vi "HV Enclosure test.vi"() -> (0 "HV Enclosure OK":bool)   [LabVIEW 2015]
uses:
  <vilib>/DAQmx/write.llb/DAQmx Write (Digital Bool 1Line 1Point).vi
  <vilib>/DAQmx/read.llb/DAQmx Read (Digital Bool 1Line 1Point).vi
  <vilib>/DAQmx/miscellaneous.llb/DAQmx Fill In Error Info.vi
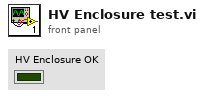
[diagram p1: front panel]
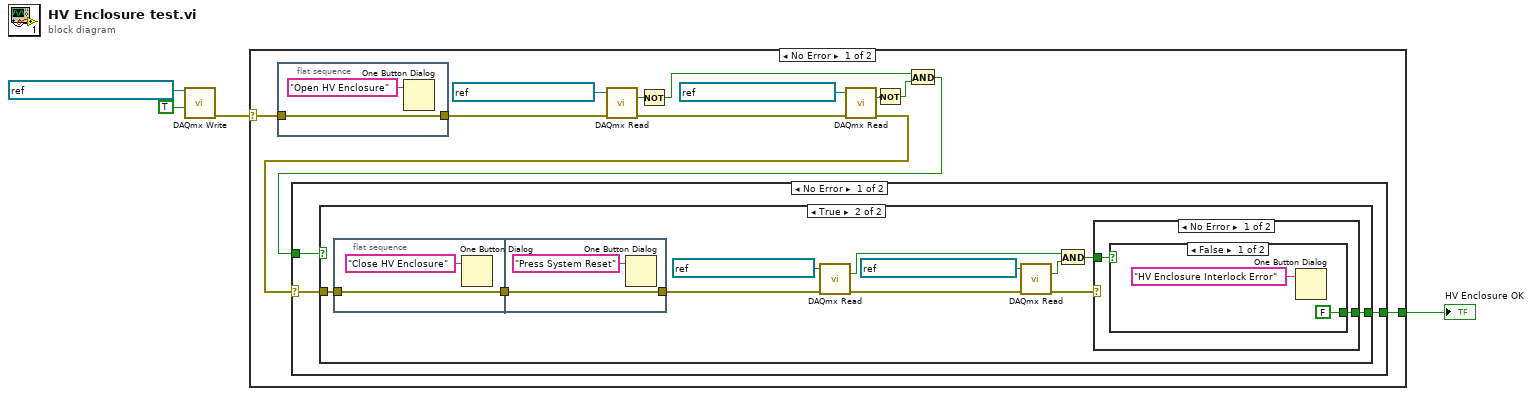
[diagram p0: block diagram]
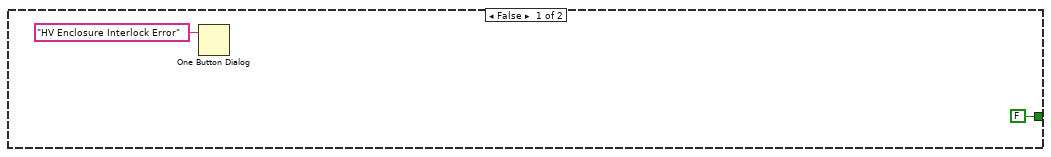
[diagram p2: hidden frame]
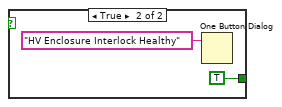
[diagram p3: hidden frame]
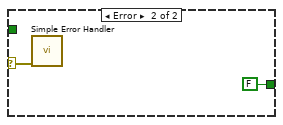
[diagram p4: hidden frame]
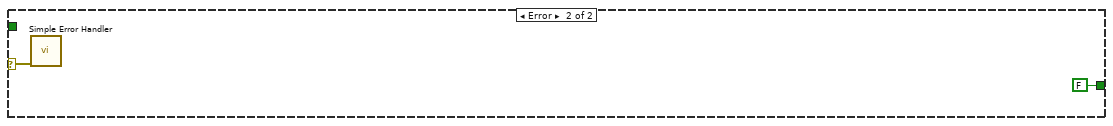
[diagram p5: hidden frame]
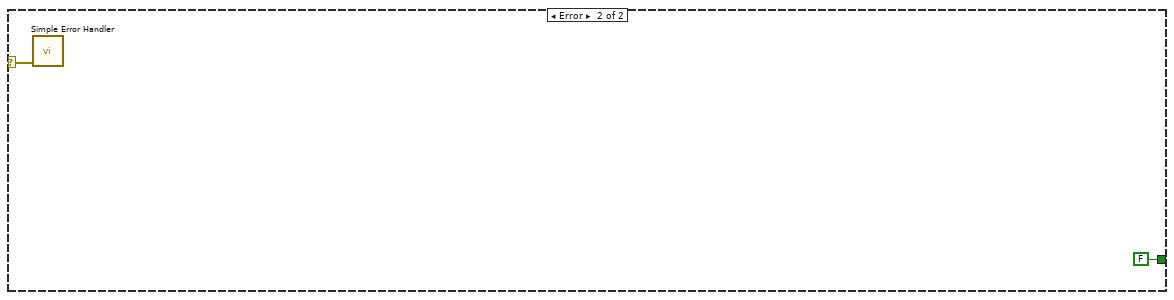
[diagram p6: hidden frame]
diagram:
  n1 = call-poly <vilib>:"DAQmx Write.vi"("task/channels in"=refnum<k21> "DO7 Unlock Door Request" ("DAQmx Global Channel"), "data"=TRUE) -> ("error out"=w4:errorcluster)  [unwired: 11 in, 2 out]
  n2 = case shown="No Error" w4 {
    selector: w4 -> [w8 w49]
    tunnel: [w5 FALSE] -> w1
    frame No Error {
      n3 = flat-sequence {
        tunnel: w8 -> [w47]
        tunnel: [w47] -> w14
        frame #0 {
          n4 = One Button Dialog(message="Open HV Enclosure") -> ()  [unwired: 1 in, 1 out]
        }
      }
      n5 = call-poly <vilib>:"DAQmx Read.vi"("task/channels in"=refnum<k21> "DI1 Safety System trip" ("DAQmx Global Channel"), "error in"=w14) -> ("data"=w13:bool, "error out"=w11:errorcluster)  [unwired: 11 in, 1 out]
      n6 = Not(x=w13) -> (.not. x?=w10:bool)
      n7 = call-poly <vilib>:"DAQmx Read.vi"("task/channels in"=refnum<k21> "DI5 Dump Switch mimic" ("DAQmx Global Channel"), "error in"=w11) -> ("data"=w12:bool, "error out"=w7:errorcluster)  [unwired: 11 in, 1 out]
      n8 = Not(x=w12) -> (.not. x?=w9:bool)
      n9 = And(x=w10, y=w9) -> (x .and. y?=w6:bool)
      n10 = case shown="No Error" w7 {
        selector: w7 -> [w19 w46]
        tunnel: w6 -> [w18 _]
        tunnel: [w17 FALSE] -> w5
        frame No Error {
          n11 = case shown="True" w18 {
            tunnel: w19 -> [_ w31]
            tunnel: [FALSE w22] -> w17
            frame False {
              n12 = One Button Dialog(message="HV Enclosure Interlock Error") -> ()  [unwired: 1 in, 1 out]
            }
            frame True {
              n13 = flat-sequence {
                tunnel: w31 -> [w41]
                tunnel: [w41] -> w32
                tunnel: [w44] -> w23
                tunnel: w32 -> [w44]
                frame #0 {
                  n14 = One Button Dialog(message="Close HV Enclosure") -> ()  [unwired: 1 in, 1 out]
                }
                frame #1 {
                  n15 = One Button Dialog(message="Press System Reset") -> ()  [unwired: 1 in, 1 out]
                }
              }
              n16 = call-poly <vilib>:"DAQmx Read.vi"("task/channels in"=refnum<k21> "DI1 Safety System trip" ("DAQmx Global Channel"), "error in"=w23) -> ("data"=w27:bool, "error out"=w30:errorcluster)  [unwired: 11 in, 1 out]
              n17 = call-poly <vilib>:"DAQmx Read.vi"("task/channels in"=refnum<k21> "DI5 Dump Switch mimic" ("DAQmx Global Channel"), "error in"=w30) -> ("data"=w26:bool, "error out"=w24:errorcluster)  [unwired: 11 in, 1 out]
              n18 = And(x=w27, y=w26) -> (x .and. y?=w25:bool)
              n19 = case shown="No Error" w24 {
                selector: w24 -> [_ w40]
                tunnel: w25 -> [w34 _]
                tunnel: [w33 FALSE] -> w22
                frame No Error {
                  n20 = case shown="False" w34 {
                    tunnel: [FALSE TRUE] -> w33
                    frame False {
                      n21 = One Button Dialog(message="HV Enclosure Interlock Error") -> ()  [unwired: 1 in, 1 out]
                    }
                    frame True {
                      n22 = One Button Dialog(message="HV Enclosure Interlock Healthy") -> ()  [unwired: 1 in, 1 out]
                    }
                  }
                }
                frame Error {
                  n23 = call <vilib>:"Simple Error Handler.vi"("error in (no error)"=w40) -> ()  [unwired: 4 in, 5 out]
                }
              }
            }
          }
        }
        frame Error {
          n24 = call <vilib>:"Simple Error Handler.vi"("error in (no error)"=w46) -> ()  [unwired: 4 in, 5 out]
        }
      }
    }
    frame Error {
      n25 = call <vilib>:"Simple Error Handler.vi"("error in (no error)"=w49) -> ()  [unwired: 4 in, 5 out]
    }
  }
  "HV Enclosure OK" <- w1
